vi "Send UI Send Action.vi"(7 "Message Priority (Normal)":T2=enum."Normal", 8 "error in (no error)":errorcluster, 9 "Action Data":variant, 10 "UI Actions":T1, 11 "Message Enqueuer":refnum<class "Message Enqueuer.lvclass">) -> (0 "error out":errorcluster, 3 "Message Enqueuer out":refnum<class "Message Enqueuer.lvclass">)   [LabVIEW 2020, in "Main_UI.lvlib" / "UI Send Action Msg.lvclass"]
doc: "This VI sends the message to an actor."
uses:
  UI Send Action Msg.lvclass
  <vilib>/ActorFramework/Message Enqueuer/Message Enqueuer.lvclass
  <vilib>/ActorFramework/Message Enqueuer/Message Priority.ctl
  Main_UI/UI Actions.ctl
  C:/Program Files/National Instruments/LabVIEW 2020/vi.lib/ActorFramework/Message/Message.lvclass
  UI Send Action Msg.lvclass/UI Send Action Msg.ctl
  <vilib>/ActorFramework/Message Enqueuer/Message Enqueuer.lvclass/Message Enqueuer.ctl
  <vilib>/ActorFramework/Message Priority Queue/Priority Enqueue.vi
  Main_UI/Main_UI.lvclass
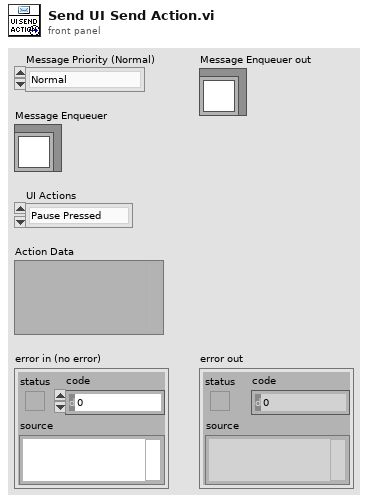
[diagram p1: front panel]
types:
  T1 = typedef "Main_UI.lvlib/Main_UI.lvclass/UI Actions.ctl" = enum16{"Pause Pressed", "Write Pressed", "RV Send Pressed", "Save Data Pressed", "Self Test Pressed", "PCRam Cell No. Changed", "Test Mode Changed"}
  T2 = typedef "Actor Framework.lvlib/Message Enqueuer.lvclass/Message Priority.ctl" = enum16{"Low", "Normal", "High"}
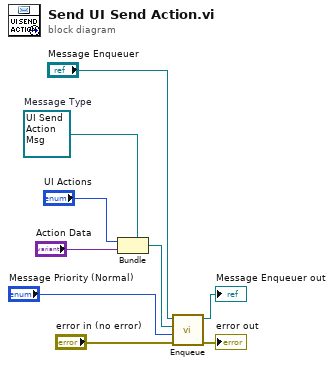
[diagram p0: block diagram]
diagram:
  w6 = refnum<class "UI Send Action Msg.lvclass"> refnum  # Message Type
  n1 = Bundle(cluster=w6, "UI Actions", "Action Data") -> (w5:refnum<class "UI Send Action Msg.lvclass">)
  n2 = call <vilib>:"Enqueue.vi"("error in (no error)"="error in (no error)", "Message Priority (Normal)"="Message Priority (Normal)", "Message"=w5, "Message Enqueuer in"="Message Enqueuer") -> ("error out"=→"error out":errorcluster, "Message Enqueuer out"=→"Message Enqueuer out":refnum<class "Message Enqueuer.lvclass">)  [unwired: 6 in]
